vi "簇转文本处理.vi"(10 "column information":T1[](array[typedef]), 11 "data":variant[](array[variant])) -> (3 "output":string)   [LabVIEW 2016]
uses:
  <vilib>/addons/database/Auxilliary.llb/DB Tools Column Info.ctl
  <vilib>/addons/database/Auxilliary.llb/DB Tools DataTypes.ctl
  <vilib>/addons/database/NI_Database_API.lvlib
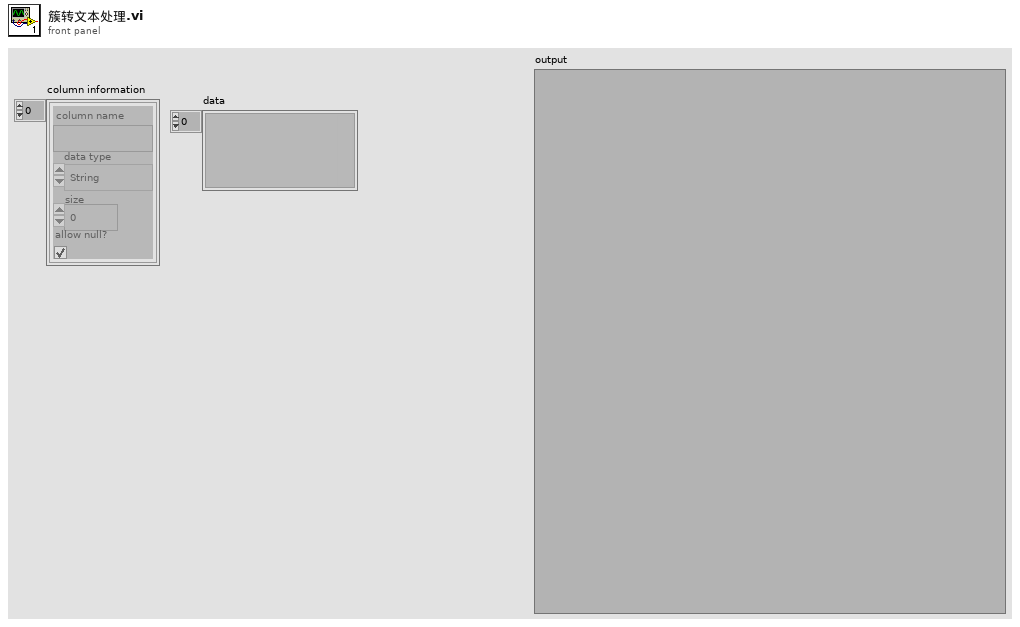
[diagram p1: front panel]
types:
  T1 = typedef "NI_Database_API.lvlib/DB Tools Column Info.ctl" = cluster{"column name":string, "data type":T2, "size":i32, "allow null?":bool}
  T2 = typedef "NI_Database_API.lvlib/DB Tools DataTypes.ctl" = enum16{"String", "Long (I32)", "Single (SGL)", "Double (DBL)", "Date/Time", "Binary"}
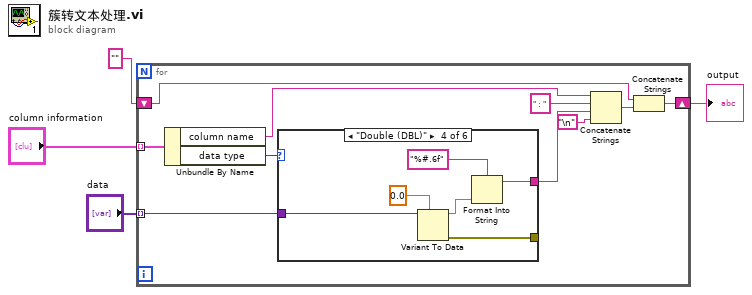
[diagram p0: block diagram]
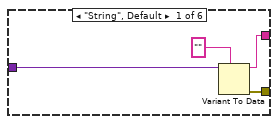
[diagram p2: hidden frame]
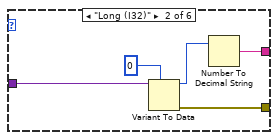
[diagram p3: hidden frame]
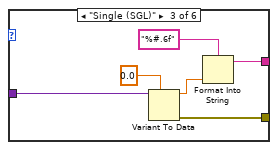
[diagram p4: hidden frame]
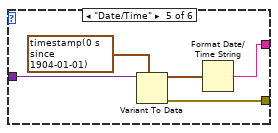
[diagram p5: hidden frame]
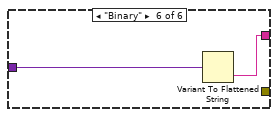
[diagram p6: hidden frame]
diagram:
  n1 = for {
    shift-right: [w10] -> w3
    shift-left: "" -> [w12]
    tunnel: "column information" -> [w9] mode=indexing
    tunnel: "data" -> [w5] mode=indexing
    n2 = Unbundle By Name(w9) -> ("column name"=w7:string, "data type"=w8:T2)
    n3 = case shown="\"Double (DBL)\"" w8 {
      tunnel: w5 -> [w17 w23 w28 w34 w40 w42]
      tunnel: [w15 w19 w27 w33 w38 _] -> _
      tunnel: [w16 w20 w24 w31 w36 w41] -> w6
      frame "String", Default {
        n4 = Variant To Data(type="", Variant=w17) -> (data=w16:string, error out=w15:errorcluster)  [unwired: 1 in]
      }
      frame "Long (I32)" {
        n5 = Variant To Data(type=0, Variant=w23) -> (data=w21:i32, error out=w19:errorcluster)  [unwired: 1 in]
        n6 = Number To Decimal String(number=w21) -> (decimal integer string=w20:string)  [unwired: 1 in]
      }
      frame "Single (SGL)" {
        n7 = Variant To Data(type=sgl 0.0, Variant=w28) -> (data=w26:sgl, error out=w27:errorcluster)  [unwired: 1 in]
        n8 = Format Into String(format string="%#.6f" ("格式字符串"), w26) -> (resulting string=w24:string)  [unwired: 2 in, 1 out]
      }
      frame "Double (DBL)" {
        n9 = Variant To Data(type=0.0, Variant=w34) -> (data=w32:dbl, error out=w33:errorcluster)  [unwired: 1 in]
        n10 = Format Into String(format string="%#.6f" ("格式字符串"), w32) -> (resulting string=w31:string)  [unwired: 2 in, 1 out]
      }
      frame "Date/Time" {
        n11 = Variant To Data(type=timestamp(0 s since 1904-01-01) ("时间标识"), Variant=w40) -> (data=w37:timestamp, error out=w38:errorcluster)  [unwired: 1 in]
        n12 = Format Date/Time String(seconds (now)=w37) -> (date/time string=w36:string)  [unwired: 2 in]
      }
      frame "Binary" {
        n13 = Variant To Flattened String(Variant=w42) -> (data string=w41:string)  [unwired: 1 out]
      }
    }
    n14 = Concatenate Strings(w7, "：" ("字符串"), w6, "\n") -> (w11:string)
    n15 = Concatenate Strings(w12, w11) -> (w10:string)
  }
  "output" <- w3
